vi "Get Deployment Target List.vi"() -> ()   [LabVIEW 2014]
panel:
  in  "Session in (localhost)":refnum<k21>="localhost" caption="Session"
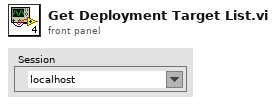
[diagram p1: front panel]
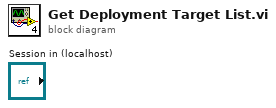
[diagram p0: block diagram]
diagram:
